vi "Detect Header.vi"(11 "input data":bool[](array[boolean])) -> (1 "header detected":bool, 2 "timestamp":u64, 3 "chdr_header":T1)   [LabVIEW 2023, in "CHDR Support.lvlib"]
doc: "Determines valid headers based on 256-bit CHDR header packet layout:\n\nConfirms valid PktType (supports 6 and 7 - Data Packet with or without a Timestamp).\nChecks for non-zero packet Length.\nChecks for expected 128 reserved bits that should always be false."
uses:
  CHDR Support.lvlib
  CHDR Header Layout.ctl
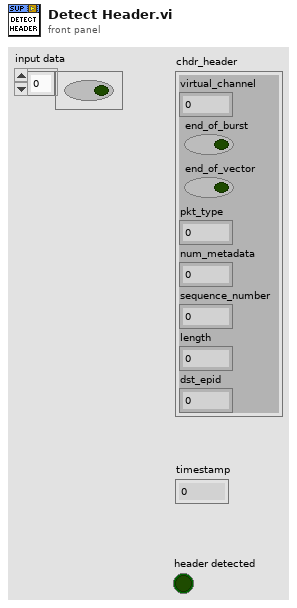
[diagram p1: front panel]
types:
  T1 = typedef "CHDR Support.lvlib/CHDR Header Layout.ctl" = cluster{"virtual_channel":fxp<+,6,6>, "end_of_burst":bool, "end_of_vector":bool, "pkt_type":fxp<+,3,3>, "num_metadata":fxp<+,5,5>, "sequence_number":u16, "length":u16, "dst_epid":u16}
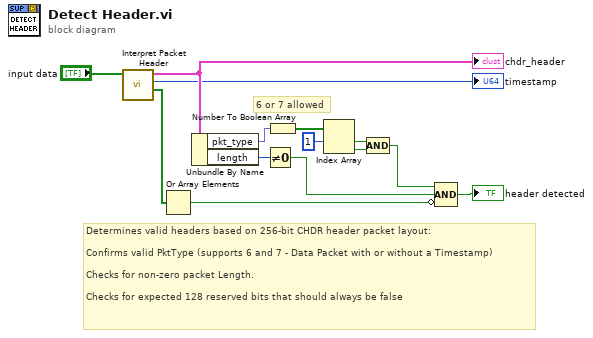
[diagram p0: block diagram]
diagram:
  # "Determines valid headers based on 256-bit CHDR header packet layout:\n\nConfirms valid PktType (supports 6 and 7 - Data Packet with or without a Timestamp)\n\nChecks for non-zero packet Length.\n\nChecks for expected 128 reserved bits that should always be false"
  # "6 or 7 allowed"
  n1 = call "Interpret Packet Header.vi"("input data"="input data") -> ("reserved_bits"=w11:bool[], "timestamp"=→"timestamp":u64, "chdr_header"=w9:T1)  [unwired: 8 in]
  "chdr_header" <- w9
  n2 = Or Array Elements(Boolean array=w11) -> (logical OR=w4:bool)
  n3 = Unbundle By Name(w9) -> ("pkt_type"=w12:fxp<+,3,3>, "length"=w10:u16)
  n4 = Not Equal To 0?(x=w10) -> (x != 0?=w5:bool)
  n5 = Number To Boolean Array(number=w12) -> (Boolean array=w13:bool[])
  n6 = Index Array(array=w13, index #1=1 ("index")) -> (element #1=w2:bool, element #2=w14:bool)  [unwired: 1 in]
  n7 = Compound Arithmetic op=AND(w2, w14) -> (w6:bool)
  n8 = Compound Arithmetic op=AND(w6, w5, invert w4) -> (→"header detected":bool)
